vi "FileSystem DEMO.vi"() -> ()   [LabVIEW 2011]
uses:
  FileSystem/FileSystem.lvclass
panel:
  out "error out":errorcluster caption="错误输出"
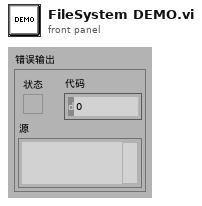
[diagram p1: front panel]
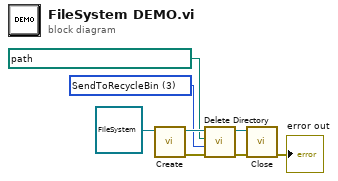
[diagram p0: block diagram]
diagram:
  w4 = 3 items=["DeletePermanently"=2, "SendToRecycleBin"=3] ("recycle")
  n1 = call "Create.vi"("FileSystem 输入"=refnum<class "FileSystem.lvclass"> refnum ("FileSystem.lvclass")) -> ("error out"=w6:errorcluster, "FileSystem 输出"=w7:refnum<class "FileSystem.lvclass">)  [unwired: 9 in]
  n2 = call "Delete Directory.vi"("error in (no error)"=w6, "recycle"=w4, "Path"=path "D:/My Documents/新建文件夹", "FileSystem 输入"=w7) -> ("error out"=w2:errorcluster, "FileSystem 输出"=w3:refnum<class "FileSystem.lvclass">)  [unwired: 6 in]
  n3 = call "Close.vi"("error in (no error)"=w2, "FileSystem 输入"=w3) -> ("error out"=→"error out":errorcluster)  [unwired: 8 in, 1 out]
